vi "Temperature converter.vi"() -> ()   [LabVIEW 2014]
panel:
  in  "Conversion":T1(ring)
  out "conerted Temp":dbl
  in  "temp C":dbl
  in  "temp F":dbl
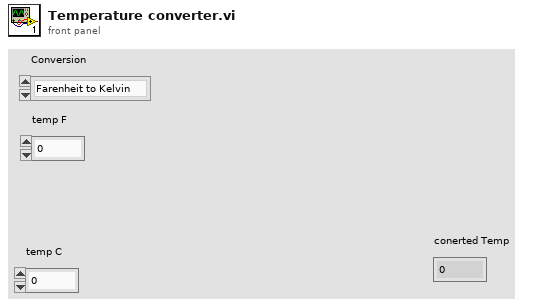
[diagram p1: front panel]
types:
  T1 = enum16{"Farenheit to Kelvin", "Celsius to Kelvin", "Farenheit to Celsius", "Celsius to Farenheit"}
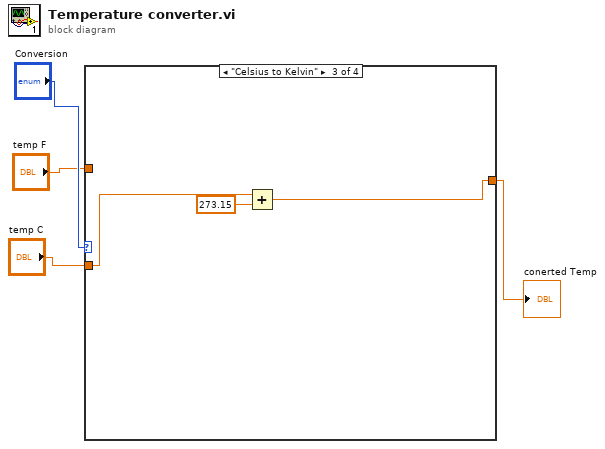
[diagram p0: block diagram]
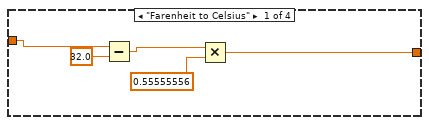
[diagram p2: hidden frame]
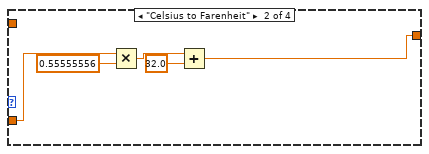
[diagram p3: hidden frame]
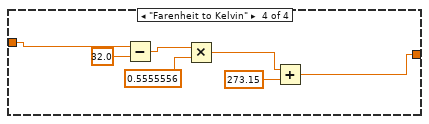
[diagram p4: hidden frame]
diagram:
  n1 = case shown="\"Celsius to Kelvin\"" "Conversion" {
    tunnel: "temp C" -> [_ w14 w17 _]
    tunnel: "temp F" -> [w9 _ _ w24]
    tunnel: [w5 w10 w15 w18] -> w1
    frame "Farenheit to Celsius" {
      n2 = Subtract(x=w9, y=32.0) -> (x-y=w7:dbl)
      n3 = Multiply(x=w7, y=0.55555556) -> (x*y=w5:dbl)
    }
    frame "Celsius to Farenheit" {
      n4 = Multiply(x=w14, y=0.55555556) -> (x*y=w12:dbl)
      n5 = Add(x=w12, y=32.0) -> (x+y=w10:dbl)
    }
    frame "Celsius to Kelvin" {
      n6 = Add(x=w17, y=273.15) -> (x+y=w15:dbl)
    }
    frame "Farenheit to Kelvin" {
      n7 = Subtract(x=w24, y=32.0) -> (x-y=w22:dbl)
      n8 = Multiply(x=w22, y=0.5555556) -> (x*y=w20:dbl)
      n9 = Add(x=w20, y=273.15) -> (x+y=w18:dbl)
    }
  }
  "conerted Temp" <- w1
